vi "Task.vi"() -> ()   [LabVIEW 2015]
uses:
  TASK ERL/List of robots.ctl
  TASK ERL/Status task.ctl
  Zmienne/common msg from UAV-1.vi
  Zmienne/common msg.vi
  Zmienne/Lokalizacja GPS/longitude Quadron.vi
  Zmienne/Lokalizacja GPS/latitude Quadron.vi
  Zmienne/Lokalizacja GPS/latitude.vi
  Zmienne/Lokalizacja GPS/longitude.vi
  Zmienne/Lokalizacja GPS/Longitude Sparus.vi
  Zmienne/Lokalizacja GPS/Latitude Sparus.vi
  Zmienne/Lokalizacja GPS/Latitude dron 1.vi
  Zmienne/Lokalizacja GPS/Longitude dron 1.vi
  Zmienne/Lokalizacja GPS/Longitude dron 2.vi
  Zmienne/Lokalizacja GPS/Latitude dron 2.vi
  TASK ERL/task erl.lvlib
  Zmienne/Lokalizacja GPS/Lokalizacja GPS.lvlib
  <vilib>/Intelligent Energy/WebSockets API/WebSockets/WebSockets.lvlib
  KML/KML.lvlib
  <vilib>/Utility/miscctls.llb/LVStringsAndValuesArrayTypeDef_U16.ctl
  Zmienne/Zmienne.lvlib
panel:
  out "nowa wiadomość":bool
  in  "Tab Control":enum32{"Drone 1", "Sparus"}(tab)
  out "error out 5":errorcluster
  out "sent messages  2":T1
  in  "ROSB WRITE 2":bool
  in  "advertise msg 3":string="{\"op\":\"advertise\", \"topic\":\"common\",\"type\":\"common_msgs/Common\"}"
  in  "rosbridge port 3":u16=9090
  in  "rosbridge server IP 3":string="192.168.1.106"
  out "raw frame 5":string="{\"op\":\"\",\"topic\":\"\",\"Msg\":{\"Sender_name\":\"Raptor\",\"Receiver_name\":\"UGV1-Raptor\",\"Latitude\":0,\"Longitude\":0,\"Value_number\":1,\"status\":\"UGV1-Raptor\"}}"
  in  "STOP ROS WRITE 2":bool
  out "raw frame 4":string="{\"op\":\"\",\"topic\":\"\",\"Msg\":{\"Sender_name\":\"Raptor\",\"Receiver_name\":\"UGV1-Raptor\",\"Latitude\":0,\"Longitude\":0,\"Value_number\":1,\"status\":\"UGV1-Raptor\"}}"
  in  "STOP ROS WRITE":bool
  in  "rosbridge server IP 2":string="192.168.1.68"
  in  "rosbridge port 2":u16=9090
  in  "advertise msg 2":string="{\"op\":\"advertise\", \"topic\":\"common\",\"type\":\"common_msgs/Common\"}"
  in  "ROSB WRITE":bool
  out "error out 4":errorcluster
  out "sent messages":T1
  out "read messages from UAV-1":T1
  in  "Mode 3":bool
  in  "String":string
  in  "Pipe":i32
  out "read messages from AUV sparus":T1
  in  "receiver robot":T2="sparus"
  in  "sender robot":T2="UGV1-Raptor"
  in  "Mode 2":bool
  in  "Additional found item":string="s"
  in  "Status sent between robots":path=path "C:/Users/User/Desktop/ERL 2017/TBM1/Surowe dane/comunnication/Common messages.txt"
  in  "Object recognition":path=path "C:/Users/User/Desktop/ERL 2017/TBM1/Surowe dane/Object recognition/object recognition.txt"
  in  "target ID":string="s"
  in  "... .jpg":string="s"
  in  "found":bool=TRUE
  in  "OPI to find":u16(ring)=3 items=["Underwater - 1 plume (made of 5 orange buoys)"=1, "Underwater - 1 pipe leaks"=2, "Underwater - debris (4 objects)"=3, "Underwater - 1 gate (made of 2 orange buoys)"=4, "Outdoor - 1 Pipe leak on land"=5, "Outdor - second damages on the building wall"=6, "Outdoor - third damages on the building wall"=7, "Indoor - 1 machine room entrance"=8, "Indoor - 1 correct valve (of four valves)"=9]
  out "OPI found":string[][](table)=[["2017-09-19T00:43:17Z", "s", "0,000000", "0,000000", "s", "UGV1-Raptor"], ["2017-09-19T00:43:22Z", "s", "0,000000", "0,000000", "s", "UGV1-Raptor"]]
  in  "Status":T2="Attached"
  in  "Additional status":string="Underwater - debris (4 objects)"
  in  "List of robots":T2="UAV-1"
  in  "Delete":bool
  in  "Number registered subtask":u16(ring)=11 items=["1"=1, "3"=2, "3"=3, "4"=4]
  out "Subtask to do":string[][](table)=[["1", "A1: Outdoors", "", "From the starting point of the building, a ground robot reaches WP5 L within a precision of 3m\navoiding obstacles along the route.", " "], ["2", "A1: Outdoors", "", "A ground robot reaches WP6 L within a precision of 3m with autonomous navigation, avoiding\nobstacles along the route. ", ""], ["3", "A1: Outdoors", "", "The robots recognise the damages outside the building (1 achievement for damage – each damage\ncan only be scored once).", ""], ["4", "A1: Outdoors", "", "The ground robot(s) build(s) an outdoor map of the land pipes area.", ""], ["5", "A1: Outdoors", "", "A ground robot detects the leak marker on the pipe.", ""], ["6", "A1: Outdoors", "", "A ground robot reports which pipe is leaking on land.", ""], ["7", "A1: Outdoors", "", "A ground robot recognises the number on the leaking pipe on land. ", ""], ["8", "A1: Outdoors", "", "Robots localise the unobstructed entrance in real-time in automatic way.", ""], ["9", "A2: Indoors", "", "A ground robot enters inside the building through the unblocked entrance.", ""], ["10", "A2: Indoors", "", "A ground robot finds a safe and unobstructed path to the machine room. (The safe path - collision\nfree from obstacles and structures - from the building entrance to the machine room must be\nshowed on the map).", ""], ["11", "A2: Indoors", "", "The ground robot(s) build a geometric indoor map of the building (Area1). ", ""], ["12", "A2: Indoors", "", "The ground robot(s) build a geometric indoor map of the building (Area2). ", ""], ["13", "A2: Indoors", "", "A ground robot recognises the machine room sign in real-time in automatic way.", ""], ["14", "A2: Indoors", "", "A ground robot enters the machine room", ""], ["15", "A2: Indoors", "", "The ground robot recognises the ID of the correct set of valves in the machine room", ""], ["16", "A2: Indoors", "", "The ground robot closes the correct valve. The robot must close one valve of the set\nautonomously and the other one manually. The process must be recorded by the on board camera\nof the robot.", ""], ["17", "A3: Underwater", "", "The underwater robot provides acoustic and optical images of the gate.", ""], ["18", "A3: Underwater", "", "The underwater robot passes through the gate without touching it. ", ""], ["19", "A3: Underwater", "", "The underwater robot passes through the gate within the first 30 minutes from the start of the run. ", ""], ["20", "A3: Underwater", "", "The underwater robot detects the five plume buoys in real time. Images are needed. ", ""], ["21", "A3: Underwater", "", "The underwater robot recognises the number on the five plume buoys. ", ""], ["22", "A3: Underwater", "", "The underwater robot produces a geometric map of the plume (Area: B1+B2). Father area from\nthe piping assembly", ""], ["23", "A3: Underwater", "", "The underwater robot produces a geometric map of the plume (Area: B3+B4+B5). Closer area to\nthe pipping assembly", ""], ["24", "A3: Underwater", "", "The underwater robot inspects the 4 pipes underwater. ", ""], ["25", "A3: Underwater", "", "The underwater robot detects the leak marker on the pipe in real time. ", ""], ["26", "A3: Underwater", "", "The underwater robot reports which is the number of the leaking pipe by its geometric position. ", ""], ["27", "A3: Underwater", "", "The underwater robot recognises and provides images of the black number stamped on the leaking\npipe", ""], ["28", "A3: Underwater", "", "Following the leaking pipe up to the assembly structure, the underwater robot provides an image\nmosaic of the first half of the leaking pipe. ", ""], ["29", "A3: Underwater", "", "Following the leaking pipe up to the assembly structure, the underwater robot provides an image\nmosaic of the second half of the leaking pipe. ", ""], ["30", "A3: Underwater", "", "The underwater robot provides a 3D reconstruction of the manipulation console where the correct\nunderwater valve is. ", ""], ["31", "A3: Underwater", "", "The underwater robot closes the correct valve with a rotation of the first 45 degrees. The process\nmust be recorded by the on board camera of the robot. ", ""], ["32", "A3: Underwater", "", "The underwater robot closes the correct valve with a rotation of the last 45 degrees (the process\nmust be recorded by the on board camera of the robot).", ""], ["33", "A4: Cooperation", "", "The underwater robot communicates through a surface robot or directly to the ground robot the\nfound leaking pipe.", ""], ["34", "A4: Cooperation", "", "The ground robot receives and decodes the message with the correct leaking pipe sent by directly\nby the underwater or through the surface robot. ", ""], ["35", "A4: Cooperation", "", "The ground robot communicates the correct land leaking pipe to the underwater robot (directly or\nthrough the surface robot). ", ""], ["36", "A4: Cooperation", "", "The underwater robot receives and decodes the message with the correct land leaking pipe sent by\nthe ground robot or the surface robot", ""], ["37", "A4: Cooperation", "", "The ground robot and the underwater robot close the correct valves in a synchronised process.", ""]]
  in  "Add leaking pipe":bool
  out "Status sent between robots and control station":string[][](table)
  in  "Cancel":bool
  in  "Setup":bool=TRUE
  in  "Done":bool=TRUE
  in  "Start":bool=TRUE
  in  "Ready":bool
  in  "stop":bool=TRUE
  out "Subtask registered event":string[][](table)
  in  "Subtask":u16(ring)=2
  out "All Subtask Status":string[][](table)=[["1", "A1: Outdoors", "", "From the starting point of the building, a ground robot reaches WP5 L within a precision of 3m\navoiding obstacles along the route.", " "], ["2", "A1: Outdoors", "", "A ground robot reaches WP6 L within a precision of 3m with autonomous navigation, avoiding\nobstacles along the route. ", ""], ["3", "A1: Outdoors", "", "The robots recognise the damages outside the building (1 achievement for damage – each damage\ncan only be scored once).", ""], ["4", "A1: Outdoors", "", "The ground robot(s) build(s) an outdoor map of the land pipes area.", ""], ["5", "A1: Outdoors", "", "A ground robot detects the leak marker on the pipe.", ""], ["6", "A1: Outdoors", "", "A ground robot reports which pipe is leaking on land.", ""], ["7", "A1: Outdoors", "", "A ground robot recognises the number on the leaking pipe on land. ", ""], ["8", "A1: Outdoors", "", "Robots localise the unobstructed entrance in real-time in automatic way.", ""], ["9", "A2: Indoors", "", "A ground robot enters inside the building through the unblocked entrance.", ""], ["10", "A2: Indoors", "", "A ground robot finds a safe and unobstructed path to the machine room. (The safe path - collision\nfree from obstacles and structures - from the building entrance to the machine room must be\nshowed on the map).", ""], ["11", "A2: Indoors", "", "The ground robot(s) build a geometric indoor map of the building (Area1). ", ""], ["12", "A2: Indoors", "", "The ground robot(s) build a geometric indoor map of the building (Area2). ", ""], ["13", "A2: Indoors", "", "A ground robot recognises the machine room sign in real-time in automatic way.", ""], ["14", "A2: Indoors", "", "A ground robot enters the machine room", ""], ["15", "A2: Indoors", "", "The ground robot recognises the ID of the correct set of valves in the machine room", ""], ["16", "A2: Indoors", "", "The ground robot closes the correct valve. The robot must close one valve of the set\nautonomously and the other one manually. The process must be recorded by the on board camera\nof the robot.", ""], ["17", "A3: Underwater", "", "The underwater robot provides acoustic and optical images of the gate.", ""], ["18", "A3: Underwater", "", "The underwater robot passes through the gate without touching it. ", ""], ["19", "A3: Underwater", "", "The underwater robot passes through the gate within the first 30 minutes from the start of the run. ", ""], ["20", "A3: Underwater", "", "The underwater robot detects the five plume buoys in real time. Images are needed. ", ""], ["21", "A3: Underwater", "", "The underwater robot recognises the number on the five plume buoys. ", ""], ["22", "A3: Underwater", "", "The underwater robot produces a geometric map of the plume (Area: B1+B2). Father area from\nthe piping assembly", ""], ["23", "A3: Underwater", "", "The underwater robot produces a geometric map of the plume (Area: B3+B4+B5). Closer area to\nthe pipping assembly", ""], ["24", "A3: Underwater", "", "The underwater robot inspects the 4 pipes underwater. ", ""], ["25", "A3: Underwater", "", "The underwater robot detects the leak marker on the pipe in real time. ", ""], ["26", "A3: Underwater", "", "The underwater robot reports which is the number of the leaking pipe by its geometric position. ", ""], ["27", "A3: Underwater", "", "The underwater robot recognises and provides images of the black number stamped on the leaking\npipe", ""], ["28", "A3: Underwater", "", "Following the leaking pipe up to the assembly structure, the underwater robot provides an image\nmosaic of the first half of the leaking pipe. ", ""], ["29", "A3: Underwater", "", "Following the leaking pipe up to the assembly structure, the underwater robot provides an image\nmosaic of the second half of the leaking pipe. ", ""], ["30", "A3: Underwater", "", "The underwater robot provides a 3D reconstruction of the manipulation console where the correct\nunderwater valve is. ", ""], ["31", "A3: Underwater", "", "The underwater robot closes the correct valve with a rotation of the first 45 degrees. The process\nmust be recorded by the on board camera of the robot. ", ""], ["32", "A3: Underwater", "", "The underwater robot closes the correct valve with a rotation of the last 45 degrees (the process\nmust be recorded by the on board camera of the robot).", ""], ["33", "A4: Cooperation", "", "The underwater robot communicates through a surface robot or directly to the ground robot the\nfound leaking pipe.", ""], ["34", "A4: Cooperation", "", "The ground robot receives and decodes the message with the correct leaking pipe sent by directly\nby the underwater or through the surface robot. ", ""], ["35", "A4: Cooperation", "", "The ground robot communicates the correct land leaking pipe to the underwater robot (directly or\nthrough the surface robot). ", ""], ["36", "A4: Cooperation", "", "The underwater robot receives and decodes the message with the correct land leaking pipe sent by\nthe ground robot or the surface robot", ""], ["37", "A4: Cooperation", "", "The ground robot and the underwater robot close the correct valves in a synchronised process.", ""]]
  in  "Subtask registered eveny":path=path "C:/Users/User/Desktop/ERL 2017/TBM1/Surowe dane/Subtask registered event.txt"
  in  "Mode":bool
  # "Manual"
  # "Autonomous"
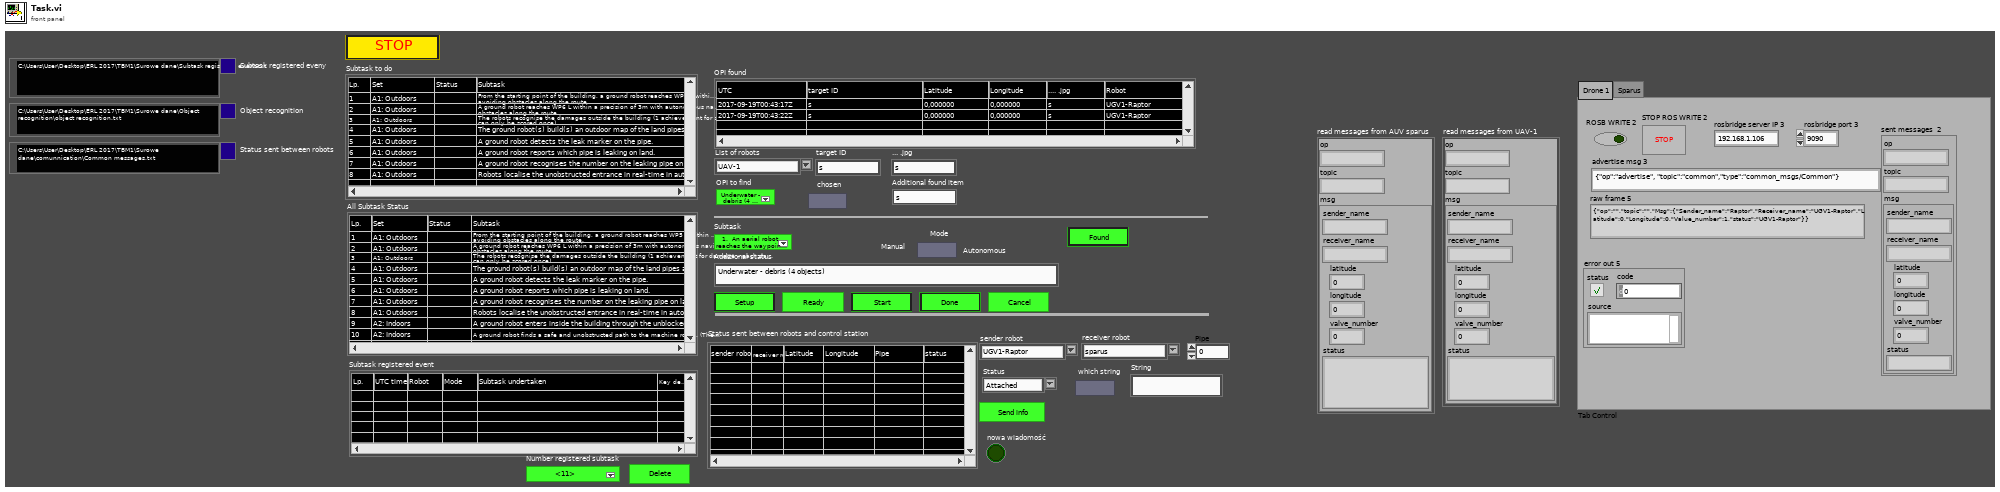
[diagram p1: front panel]
types:
  T1 = cluster{"op":string, "topic":string, "msg":cluster{"sender_name":string, "receiver_name":string, "latitude":dbl, "longitude":dbl, "valve_number":i32, "status":string}}
  T2 = typedef "Biblioteka moduł map v3.lvlib/task erl.lvlib/List of robots.ctl" = string
  T3 = cluster{"AUV-Sparus":cluster{"Navigation data":string[][], "Data sampling frequency":string}, "UAV-1":cluster{"Navigation data":string[][], "Data sampling frequency":string}, "UAV-2":cluster{"Navigation data":string[][], "Data sampling frequency":string}, "UGV1-Raptor":cluster{"Navigation data":string[][], "Data sampling frequency":string}, "UGV2-Quadron":cluster{"Navigation data":string[][], "Data sampling frequency":string}}
  T4 = typedef "LVStringsAndValuesArrayTypeDef_U16.ctl" = cluster{"String":string, "Value":u16}[]
  T5 = typedef "Biblioteka moduł map v3.lvlib/task erl.lvlib/Status task.ctl" = string
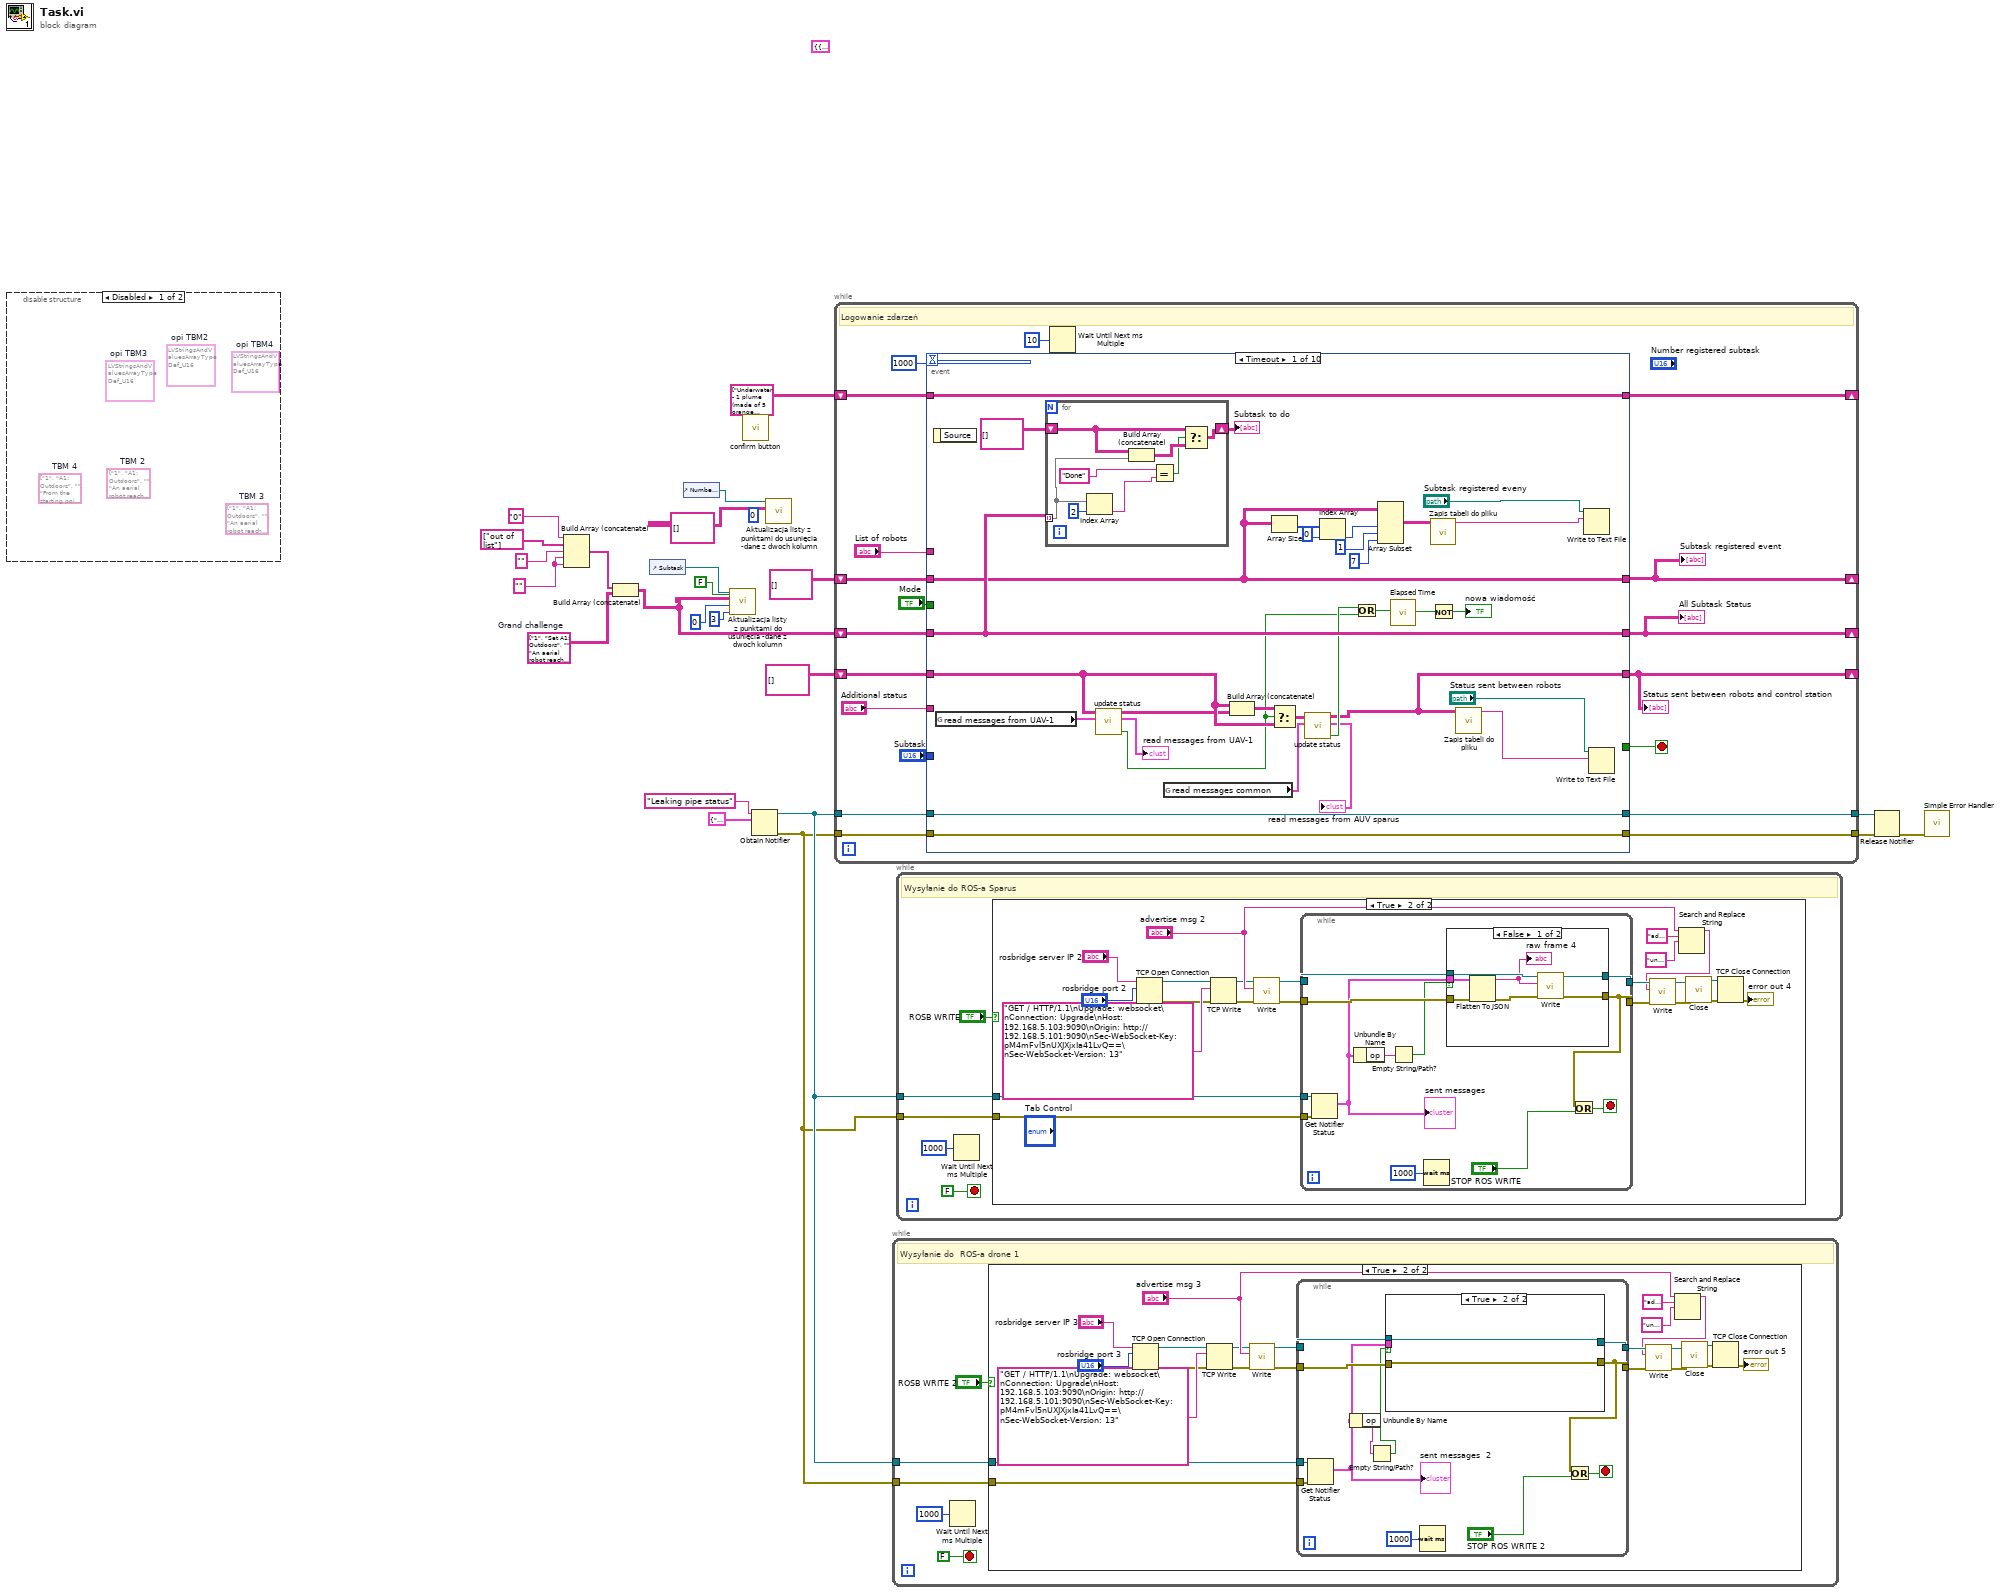
[diagram p0: block diagram]
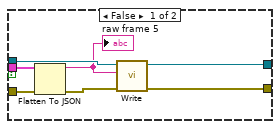
[diagram p3: hidden frame]
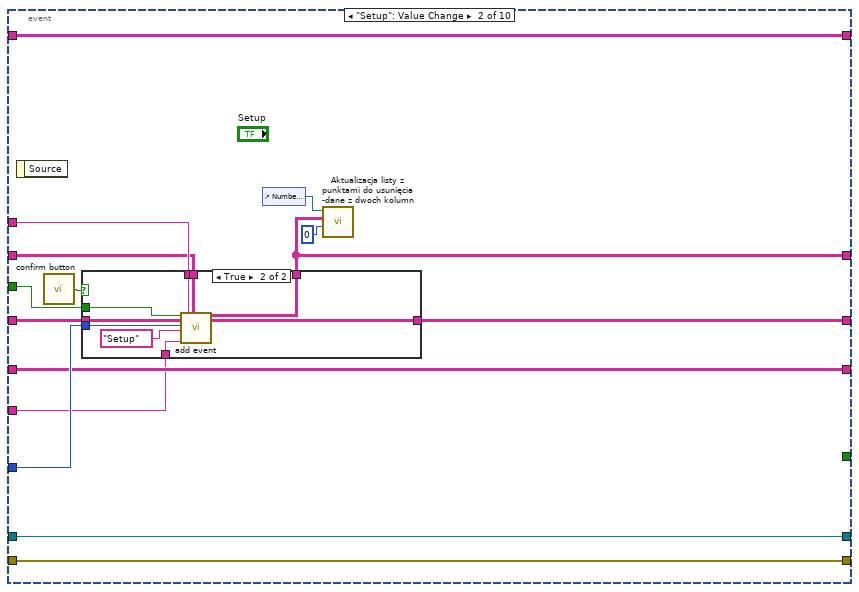
[diagram p7: hidden frame]
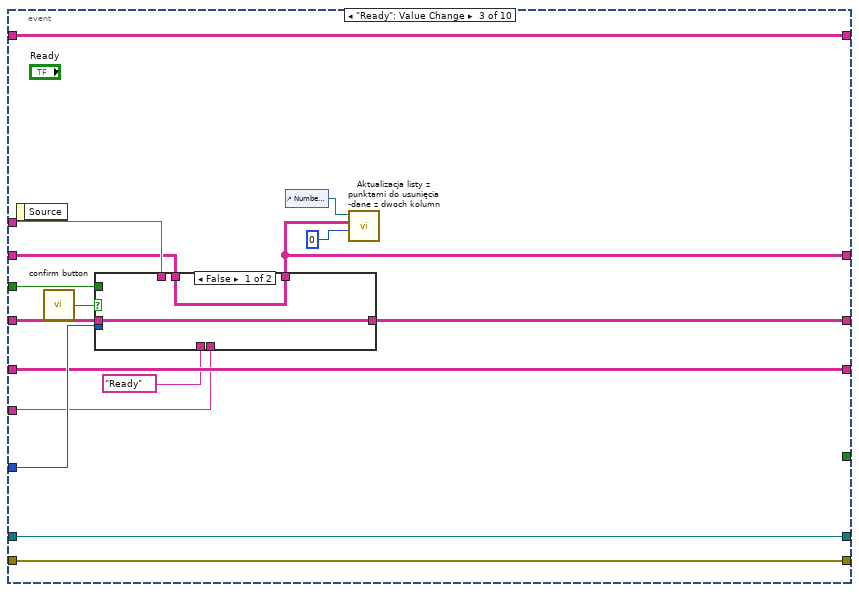
[diagram p9: hidden frame]
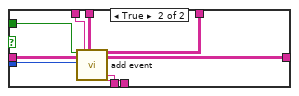
[diagram p10: hidden frame]
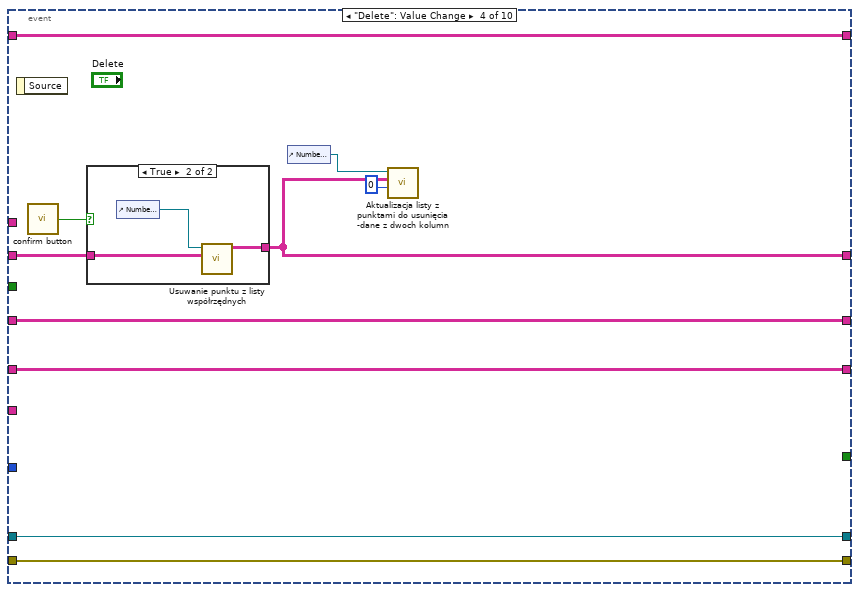
[diagram p11: hidden frame]
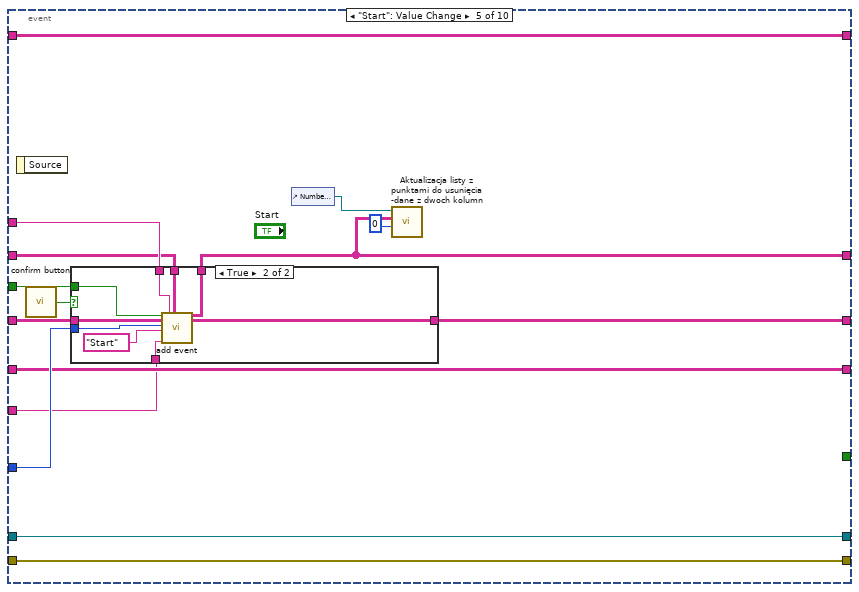
[diagram p13: hidden frame]
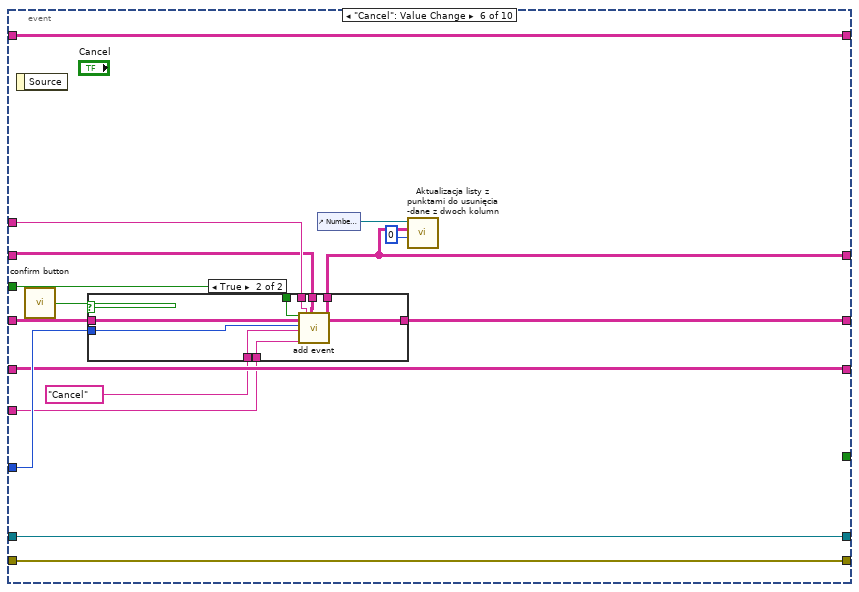
[diagram p15: hidden frame]
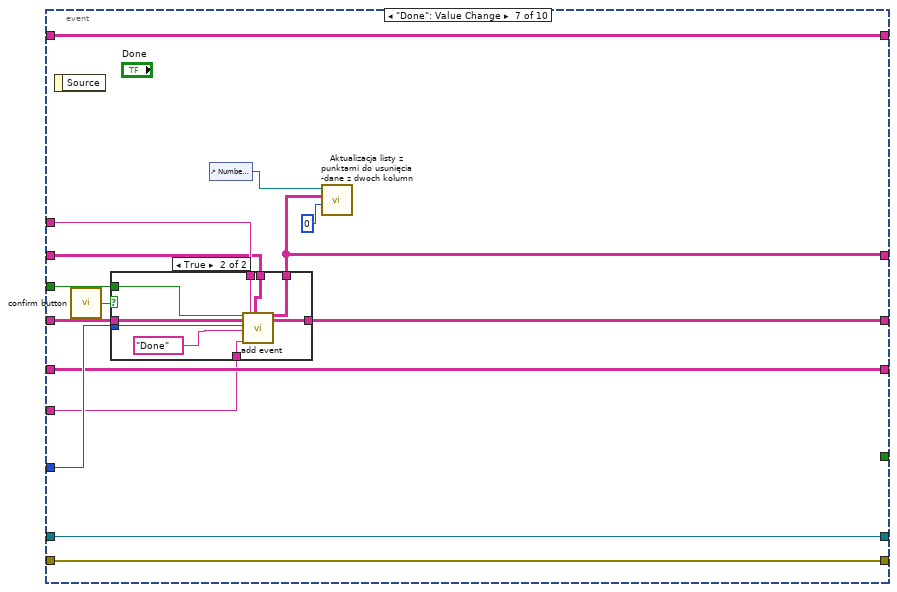
[diagram p17: hidden frame]
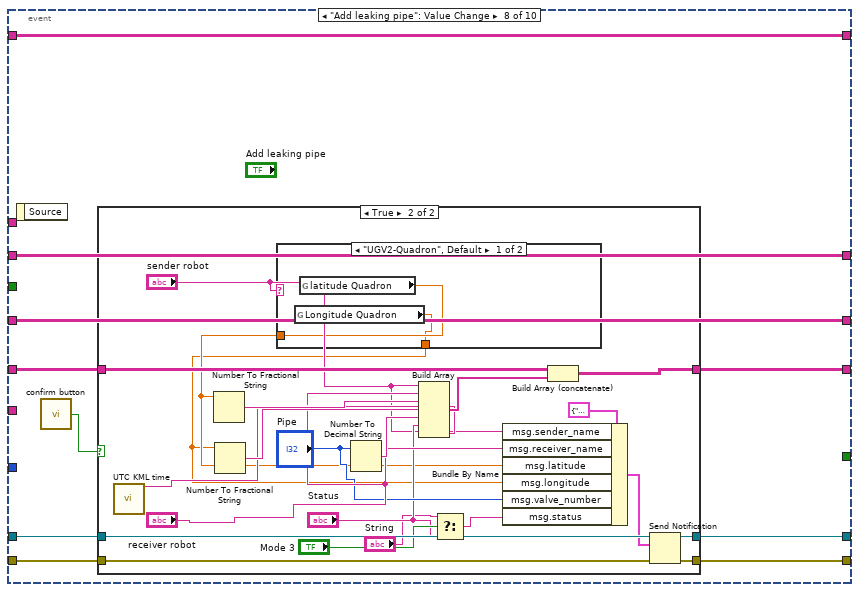
[diagram p19: hidden frame]
diagram:
  w3 = string[][] [["1", "Set A1: Outdoors", "", "An aerial robot reaches the waypoints WP1 A within a radius of 5 m in autonomous navigation."], ["2", "Set A1: Outdoors", "", "An aerial robot reaches the waypoints WP2 A within a radius of 5 m in autonomous navigation."], ["3", "Set A1: Outdoors", "", "An aerial robot reaches the waypoints WP3 A within a radius of 5 m in autonomous navigation."], ["4", "Set A1: Outdoors", "", "A ground robot reaches the waypoints WP1 L within a precision of 3m."], ["5", "Set A1: Outdoors", "", "A ground robot reaches the waypoints WP2 L within a precision of 3m."], ["6", "Set A1: Outdoors", "", "A ground robot reaches the waypoints WP5 L within a precision of 3m."], ["7", "Set A1: Outdoors", "", "A ground robot reaches the WP3 L within a precision of 3 m in autonomous navigation."], ["8", "Set A1: Outdoors", "", "A ground robot reaches the WP4 L within a precision of 3 m in autonomous navigation."], ["9", "Set A1: Outdoors", "", "A ground robot reaches the WP6 L within a precision of 3 m in autonomous navigation."], ["10", "Set A1: Outdoors", "", "Within 30 minutes of start of the run, a robot reports the correct location (within radius 5 m) of the missing worker outside the building. "], ["11", "Set A1: Outdoors", "", "An aerial robot deploys the first-aid kit (within radius 2 m) from the worker outside the building"], ["12", "Set A1: Outdoors", "", "The aerial robot transfers the first-aid kit to the land robot outside the building. (It must be directly deployed on the platform or within a radius of 1 m from it) "], ["13", "Set A1: Outdoors", "", "Robots reports the damages on the land pipes. D1"], ["14", "Set A1: Outdoors", "", "Robots reports the damages on the land pipes. D2"], ["15", "Set A1: Outdoors", "", "Robots reports the damages on the land pipes. D3"], ["16", "Set A1: Outdoors", "", "A robot detects the leak marker on the pipe."], ["17", "Set A1: Outdoors", "", "A robot reports the pipe that is leaking on land. "], ["18", "Set A1: Outdoors", "", "A robot recognises the number on the leaking pipe on land. "], ["19", "Set A1: Outdoors", "", "The robots recognise the damages on the wall of the building.  D1"], ["20", "Set A1: Outdoors", "", "The robots recognise the damages on the wall of the building.  D2"], ["21", "Set A1: Outdoors", "", "The robots recognise the damages on the wall of the building.  D3"], ["22", "Set A1: Outdoors", "", "A robot localises the unobstructed entrance in real-time in automatic way."], ["23", "Set A1: Outdoors", "", "Robots localise the obstructed entrances. E1"], ["24", "Set A1: Outdoors", "", "Robots localise the obstructed entrances. E2"], ["25", "Set A1: Outdoors", "", "Robots find a safe and unobstructed path to the unblocked entry of the building for a ground robot. (The path is shown on the map). "], ["26", "Set A1: Outdoors", "", "From the starting point, a ground robot follows a safe path (collision free from obstacles and structures) to the unobstructed building entrance."], ["27", "Set A1: Outdoors", "", "The aerial robot builds a 2D or 3D map of the designated vertical wall "], ["28", "Set A1: Outdoors", "", "The aerial robot builds the map on board during the flight. The map must be shown to the referees just after the flight finishes. "], ["29", "Set A1: Outdoors", "", "Robots build an outdoor map of the land pipes area with OPIs (North-West side)."], ["30", "Set A1: Outdoors", "", "Robots build an outdoor map of the land pipes area with OPIs (North-East side)."], ["31", "Set A1: Outdoors", "", "Robots build an outdoor map of the land pipes area with OPIs (South-West side)."], ["32", "Set A1: Outdoors", "", "Robots build an outdoor map of the land pipes area with OPIs (South-East side)."], ["33", "Set A2: Indoors", "", "A ground robot enters the building through the unobstructed door"], ["34", "Set A2: Indoors", "", "Within 30 minutes of start of the run, a ground robot reports the correct location of the missing worker inside the building. "], ["35", "Set A2: Indoors", "", "The missing worker is detected in real-time in an automatic way. "], ["36", "Set A2: Indoors", "", "A ground robot deploys the first-aid kit (within radius 1 m) from the worker inside the building. \n"], ["37", "Set A2: Indoors", "", "The ground robot(s) recognise the damages on the wall of the building.  D1"], ["38", "Set A2: Indoors", "", "The ground robot(s) recognise the damages on the wall of the building.  D2"], ["39", "Set A2: Indoors", "", "From the building entrance, a ground robot follows a safe path (collision free from obstacles and structures) to the machine room. "], ["40", "Set A2: Indoors", "", "A ground robot recognises the machine room sign in real-time and in automatic way."], ["41", "Set A2: Indoors", "", "A ground robot enters the machine room. "], ["42", "Set A2: Indoors", "", "The ground robot(s) builds a geometric indoor map of the building.  Area 1"], ["43", "Set A2: Indoors", "", "The ground robot(s) builds a geometric indoor map of the building.  Area 2"], ["44", "Set A2: Indoors", "", "A ground robot recognises the ID of the correct set of valves in the machine room."], ["45", "Set A2: Indoors", "", "A ground robot closes the correct valve manual."], ["46", "Set A2: Indoors", "", "A ground robot closes the correct valve autonomous."], ["47", "Set A3: Underwater", "", "The underwater robot provides images of the gate. Acoustic buoy-1"], ["48", "Set A3: Underwater", "", "The underwater robot provides images of the gate. Acoustic buoy-2 "], ["49", "Set A3: Underwater", "", "The underwater robot provides images of the gate. Optical buoy-1"], ["50", "Set A3: Underwater", "", "The underwater robot provides images of the gate. Optical buoy-2"], ["51", "Set A3: Underwater", "", "The underwater robot detects the plume buoys in real time. Images are needed.  B1"], ["52", "Set A3: Underwater", "", "The underwater robot detects the plume buoys in real time. Images are needed.  B2"], ["53", "Set A3: Underwater", "", "The underwater robot detects the plume buoys in real time. Images are needed.  B3"], ["54", "Set A3: Underwater", "", "The underwater robot detects the plume buoys in real time. Images are needed.  B4"], ["55", "Set A3: Underwater", "", "The underwater robot detects the plume buoys in real time. Images are needed.  B5"], ["56", "Set A3: Underwater", "", "The underwater robot recognises the number on the plume buoys B1"], ["57", "Set A3: Underwater", "", "The underwater robot recognises the number on the plume buoys B2"], ["58", "Set A3: Underwater", "", "The underwater robot recognises the number on the plume buoys B3"], ["59", "Set A3: Underwater", "", "The underwater robot recognises the number on the plume buoys B4"], ["60", "Set A3: Underwater", "", "The underwater robot recognises the number on the plume buoys B5"], ["61", "Set A3: Underwater", "", "The underwater robot produces a geometric map of the plume (Area: B1+B2)."], ["62", "Set A3: Underwater", "", "The underwater robot produces a geometric map of the plume (Area: B3+B4+B5)."], ["63", "Set A3: Underwater", "", "The underwater robot detects the leak marker on the pipe in real time. "], ["64", "Set A3: Underwater", "", "The underwater robot recognises and provides images of the black number stamped on the leaking pipe."], ["65", "Set A3: Underwater", "", "The underwater robot reports which is the number of the leaking pipe by its geometric position. "], ["66", "Set A3: Underwater", "", "The underwater robot inspects the four pipes underwater. Provide images.1"], ["67", "Set A3: Underwater", "", "The underwater robot inspects the four pipes underwater. Provide images.2"], ["68", "Set A3: Underwater", "", "The underwater robot inspects the four pipes underwater. Provide images.3"], ["69", "Set A3: Underwater", "", "The underwater robot inspects the four pipes underwater. Provide images.4"], ["70", "Set A3: Underwater", "", "Following the leaking pipe up to the assembly structure, the underwater robot provides an image mosaic of the first half of the leaking pipe."], ["71", "Set A3: Underwater", "", "Following the leaking pipe up to the assembly structure, the underwater robot provides an image mosaic of the second half of the leaking pipe. "], ["72", "Set A3: Underwater", "", "The underwater robot provides images of the structure sides.  North"], ["73", "Set A3: Underwater", "", "The underwater robot provides images of the structure sides.  South"], ["74", "Set A3: Underwater", "", "The underwater robot provides images of the structure sides.  East"], ["75", "Set A3: Underwater", "", "The underwater robot provides images of the structure sides.  West"], ["76", "Set A3: Underwater", "", "The underwater robot provides a 3D reconstruction of the structure. "], ["77", "Set A3: Underwater", "", "The underwater robot localises the missing worker underwater within a radius of 5 meters."], ["78", "Set A3: Underwater", "", "The underwater robot gives the dimensions and geometrical shape of the closest object to the worker"], ["79", "Set A3: Underwater", "", "The underwater robot provides 3D reconstruction of the worker."], ["80", "Set A3: Underwater", "", "The underwater robot provides a 2D acoustic or optical map of the debris.  Area 1"], ["81", "Set A3: Underwater", "", "The underwater robot provides a 2D acoustic or optical map of the debris.  Area 2"], ["82", "Set A3: Underwater", "", "The underwater robot provides a 3D reconstruction of the manipulation console where the correct underwater valve is. "], ["83", "Set A3: Underwater", "", "The underwater robot closes the correct valve with a rotation of the first 45 degrees. The process must be recorded by the on board camera of the robot"], ["84", "Set A3: Underwater", "", "The underwater robot closes the correct valve with a rotation of the last 45 degrees.  The process must be recorded by the on board camera of the robot."], ["85", "Set A4: Cooperation", "", "The underwater robot communicates the correct underwater leaking pipe to the aerial or ground robot. Directly or through the surface robot."], ["86", "Set A4: Cooperation", "", "The aerial or ground robot receives and decodes the message with the correct leaking pipe sent by directly by the underwater or through the surface robot."], ["87", "Set A4: Cooperation", "", "The aerial or ground robot communicates the correct land leaking pipe to the underwater robot (directly or through the surface robot)."], ["88", "Set A4: Cooperation", "", "The underwater robot receives and decodes the message with the correct land leaking pipe sent by the aerial or ground robot (directly or through the surface robot)."], ["89", "Set A4: Cooperation", "", "The ground robot and the underwater robot close the correct valves in a synchronised process. "], ["90", "Set A4: Cooperation", "", "The aerial robot communicates to the ground robot the safe path to the building"], ["91", "Set A5: General", "", "The ground robots return to the landing area once all the tasks have been done"], ["92", "Set A5: General", "", "The underwater robot surfaces in a controlled way once all the tasks have been done."], ["93", "Set A5: General", "", "The aerial robots return to the landing area once all the tasks have been done. "], ["94", "Set A5: General", "", "The ground robot(s) transmits live position and images/video to the control station during the run. "], ["95", "Set A5: General", "", "The aerial robot(s) transmits live position and images/video to the control station during the run. "], ["96", "Set A5: General", "", "The marine robot(s) transmits live position and images/video to the control station during the run or the manipulation task."]]  # Grand challenge
  w10 = ""
  (unwired) T3 {"AUV-Sparus"={"Navigation data"=[], "Data sampling frequency"=""}, "UAV-1"={"Navigation data"=[], "Data sampling frequency"=""}, "UAV-2"={"Navigation data"=[], "Data sampling frequency"=""}, "UGV1-Raptor"={"Navigation data"=[], "Data sampling frequency"=""}, "UGV2-Quadron"={"Navigation data"=[], "Data sampling frequency"=""}} ("Vehicle navigation data")
  (unwired) 0 ("text add 1")
  n1 = disable-structure shown="Disabled" {
    frame Disabled {
      (unwired) string[][] [["1", "A1: Outdoors", "", "An aerial robot reaches WP1A, WP2A, WP3A, within a radius of 5 meters with autonomous\nnavigation. Waypoints can be reached in no specific order and the team can suggest additional\nwaypoints to their flight plan.", " "], ["2", "A1: Outdoors", "", "Within first 30 minutes of the start of the run, an aerial robot reports correct location (within\nradius of 5 m) of the missing worker on land.", ""], ["3", "A1: Outdoors", "", "An aerial robot deploys the first-aid kit within a radius of 2 m from the worker found on land", ""], ["4", "A1: Outdoors", "", "An aerial robot reports which pipe(s) are damaged on land (one achievement per damage).", ""], ["5", "A1: Outdoors", "", "An aerial robot detects the leak marker on the pipe.", ""], ["6", "A1: Outdoors", "", "An aerial robot reports which pipe is leaking on land", ""], ["7", "A1: Outdoors", "", "The aerial robot builds an outdoor map of the land pipes area with OPIs (North-West side). Use\nthe information from each robot to provide only one map.", ""], ["8", "A1: Outdoors", "", "The aerial robot builds an outdoor map of the land pipes area with OPIs (North-East side). Use\nthe information from each robot to provide only one map.", ""], ["9", "A1: Outdoors", "", "The aerial robot builds an outdoor map of the land pipes area with OPIs (South-West side). Use\nthe information from each robot to provide only one map.", ""], ["10", "A1: Outdoors", "", "The aerial robot builds an outdoor map of the land pipes area with OPIs (South-East side). Use\nthe information from each robot to provide only one map.", ""], ["11", "A1: Outdoors", "", "The aerial robot builds the maps on board during the flight. The maps must be shown to the\nreferees just after the flight finishes. ", ""], ["12", "Set A2: Underwater", "", "The underwater robot provides acoustic and optical images of the gate.", ""], ["13", "Set A2: Underwater", "", "The underwater robot passes through the gate without touching it. ", ""], ["14", "Set A2: Underwater", "", "The underwater robot passes through the gate within the first 30 minutes from the start of the run. ", ""], ["15", "Set A2: Underwater", "", "The underwater robot detects the five plume buoys in real time. Images are needed. ", ""], ["16", "Set A2: Underwater", "", "The underwater robot recognises the number on the five plume buoys. ", ""], ["17", "Set A2: Underwater", "", "The underwater robot produces a geometric map of the plume (Area: B1+B2). Father area from\nthe piping assembly.", ""], ["18", "Set A2: Underwater", "", "The underwater robot produces a geometric map of the plume (Area: B3+B4+B5). Closer area to\nthe pipping assembly", ""], ["19", "Set A2: Underwater", "", "The underwater robot detects the leak marker on the pipe in real time. ", ""], ["20", "Set A2: Underwater", "", "The underwater robot recognises and provides images of the black number stamped on the leaking\npipe.", ""], ["21", "Set A2: Underwater", "", "The underwater robot reports which is the number of the leaking pipe by its geometric position. ", ""], ["22", "Set A2: Underwater", "", "Following the leaking pipe up to the assembly structure, the underwater robot provides an image\nmosaic of the first half of the leaking pipe. ", ""], ["23", "Set A2: Underwater", "", "Following the leaking pipe up to the assembly structure, the underwater robot provides an image\nmosaic of the second half of the leaking pipe. ", ""], ["24", "Set A2: Underwater", "", "The underwater robot provides images of the structure sides (North, South, East and West).", ""], ["25", "Set A2: Underwater", "", "The underwater robot provides a 3D reconstruction of the structure (front and rear).", ""], ["26", "Set A2: Underwater", "", "The underwater robot provides a 2D acoustic or optical map of the debris (Area 1 and Area 2", ""], ["27", "Set A2: Underwater", "", "The underwater robot localises the missing worker underwater within a radius of 5 meters.\nProvide images and latitude/longitude.", ""], ["28", "Set A2: Underwater", "", "The underwater robot gives the dimensions and geometrical shape of the closest object to the\nworker", ""], ["29", "Set A2: Underwater", "", "The underwater robot provides 3D reconstruction of the worker.", ""], ["30", "Set A2: Underwater", "", "The underwater robot surfaces within a radius of 2 meters from the worker position.", ""], ["31", "Set A3: Cooperation", "", "The underwater robot communicates directly or through a surface robot to the aerial robot the\nposition of the underwater worker (within a radius of 5 meters).", ""], ["32", "Set A3: Cooperation", "", "The aerial robot receives and decodes the message with the position of the worker sent by the\nunderwater/surface robot.", ""], ["33", "Set A3: Cooperation", "", "The aerial robot, upon receiving the position of the underwater worker, takes a picture (from the\nauthorised aerial volume) of the harbour area showing either the underwater robot or the surface\nrobot on the position that marks where the worker is. (The image includes location).", ""], ["34", "Set A3: Cooperation", "", "The underwater robot communicates the correct underwater leaking pipe to the aerial robot. ", ""], ["35", "Set A3: Cooperation", "", "The aerial robot receives and decodes the message with the correct leaking pipe sent by directly\nby the underwater or through the surface robot. ", ""], ["36", "Set A3: Cooperation", "", "The aerial robot communicates the correct land leaking pipe to the underwater robot (directly or\nthrough the surface robot). ", ""], ["37", "Set A3: Cooperation", "", "The underwater robot receives and decodes the message with the correct land leaking pipe sent by\nthe aerial robot or the surface robot.", ""], ["38", "Set A4: General", "", "The aerial robots return to the landing area once all the tasks have been done. ", ""], ["39", "Set A4: General", "", "The underwater robot surfaces in a controlled way once all the tasks have been done.", ""], ["40", "Set A4: General", "", "Benchmarking data is delivered appropriately (time and format)", ""], ["41", "Set A4: General", "", "The aerial robot(s) transmits live position and images/video to the control station during the run", ""], ["42", "Set A4: General", "", "The marine robot(s) transmits live position and images/video to the control station during the run\nor the manipulation task.", ""]]  # TBM 3
      (unwired) string[][] [["1", "A1: Outdoors", "", "An aerial robot reaches WP1A, WP2A, WP3A, within a radius of 5 meters with autonomous\nnavigation. Waypoints can be reached in no specific order and the team can suggest additional\nwaypoints to their flight plan.", " "], ["2", "A1: Outdoors", "", "A ground robot reaches WP1L with a precision of 3 m.", ""], ["3", "A1: Outdoors", "", "A ground robot reaches WP2 L with a precision of 3 m.", ""], ["4", "A1: Outdoors", "", "A ground robot reaches WP3 L within a precision of 3 m in autonomous navigation.", ""], ["5", "A1: Outdoors", "", "A ground robot reaches land piping area WP4 L within a precision of 3 m in autonomous\nnavigation.", ""], ["6", "A1: Outdoors", "", "Within first 30 minutes of the start of the run, a robot reports correct location (within radius of 5\nm) of the missing worker outside the building.", ""], ["7", "A1: Outdoors", "", "An aerial robot deploys the first-aid kit within a radius of 2 m from the worker found on land\noutside the building.", ""], ["8", "A1: Outdoors", "", "An aerial robot transfers the first-aid kit to the land robot outside the building. (It must be directly\ndeployed on the platform or within a radius of 1 m from it).", ""], ["9", "A1: Outdoors", "", "Robots recognise the damages outside the building (1 achievement for damage – each damage can\nonly be scored once).", ""], ["10", "A1: Outdoors", "", "Robots localise the unobstructed entrance in an automatic way", ""], ["11", "A1: Outdoors", "", "Robots localise the obstructed entrances.", ""], ["12", "A1: Outdoors", "", "Robots find a safe and unobstructed path to the unblocked entry of the building for the ground\nrobot (the safe path - collision free from obstacles and structures - from the starting point to the\nunobstructed building entrance must be showed on the map).", ""], ["13", "A1: Outdoors", "", "Robots build an outdoor map of the land pipes area with OPIs (North-West side). Use the\ninformation from each domain and from each robot to provide only one map.", ""], ["14", "A1: Outdoors", "", "Robots build an outdoor map of the land pipes area with OPIs (North-East side).Use the\ninformation from each domain and from each robot to provide only one map.", ""], ["15", "A1: Outdoors", "", "Robots build an outdoor map of the land pipes area with OPIs (South-West side). Use the\ninformation from each domain and from each robot to provide only one map.", ""], ["16", "A1: Outdoors", "", "Robots build an outdoor map of the land pipes area with OPIs (South-East side).Use the\ninformation from each domain and from each robot to provide only one map.", ""], ["17", "A2: Indoors", "", "A ground robot enters the building", ""], ["18", "A2: Indoors", "", "Within first 30 minutes of the start of the run, a ground robot reports correct location of missing\nworker inside the building.", ""], ["19", "A2: Indoors", "", "The missing worker is detected in real-time in an automatic way.", ""], ["20", "A2: Indoors", "", "A ground robot deploys the first-aid kit within a radius of 1 m from the worker found inside the\nbuilding.", ""], ["21", "A2: Indoors", "", "The ground robot(s) recognise the damages inside the building (1 achievement for damage – each\ndamage can only be scored once).", ""], ["22", "A2: Indoors", "", "A ground robot finds a safe and unobstructed path to the machine room. (The safe path - collision\nfree from obstacles and structures - from the building entrance to the machine room must be\nshowed on the map).", ""], ["23", "A2: Indoors", "", "A ground robot recognizes the machine room sign in real-time and in automatic way.", ""], ["24", "A2: Indoors", "", "A ground robot enters the machine room.", ""], ["25", "A2: Indoors", "", "The ground robot(s) build a geometric indoor map of the building (Area1). (Use the best map or a\ncombination of ground robots maps)", ""], ["26", "A2: Indoors", "", "The ground robot(s) build a geometric indoor map of the building (Area2). (Use the best map or a\ncombination of ground robots maps).", ""], ["27", "A3: Cooperation", "", "The aerial robot communicates to the land robot the safe path to the building.", ""], ["28", "A4: General", "", "The aerial robots return to the landing area once all the tasks have been done. ", ""], ["29", "A4: General", "", "The ground robots return to the landing area all the tasks have been done.", ""], ["30", "A4: General", "", "Benchmarking data is delivered appropriately (time and format)", ""], ["31", "A4: General", "", "The ground robot(s) transmits live position and images/video to the control station during the run.", ""], ["32", "A4: General", "", "The aerial robot(s) transmits live position and images/video to the control station during the run.", ""]]  # TBM 2
      (unwired) string[][] [["1", "A1: Outdoors", "", "From the starting point of the building, a ground robot reaches WP5 L within a precision of 3m\navoiding obstacles along the route.", " "], ["2", "A1: Outdoors", "", "A ground robot reaches WP6 L within a precision of 3m with autonomous navigation, avoiding\nobstacles along the route. ", ""], ["3", "A1: Outdoors", "", "The robots recognise the damages outside the building (1 achievement for damage – each damage\ncan only be scored once).", ""], ["4", "A1: Outdoors", "", "The ground robot(s) build(s) an outdoor map of the land pipes area.", ""], ["5", "A1: Outdoors", "", "A ground robot detects the leak marker on the pipe.", ""], ["6", "A1: Outdoors", "", "A ground robot reports which pipe is leaking on land.", ""], ["7", "A1: Outdoors", "", "A ground robot recognises the number on the leaking pipe on land. ", ""], ["8", "A1: Outdoors", "", "Robots localise the unobstructed entrance in real-time in automatic way.", ""], ["9", "A2: Indoors", "", "A ground robot enters inside the building through the unblocked entrance.", ""], ["10", "A2: Indoors", "", "A ground robot finds a safe and unobstructed path to the machine room. (The safe path - collision\nfree from obstacles and structures - from the building entrance to the machine room must be\nshowed on the map).", ""], ["11", "A2: Indoors", "", "The ground robot(s) build a geometric indoor map of the building (Area1). ", ""], ["12", "A2: Indoors", "", "The ground robot(s) build a geometric indoor map of the building (Area2). ", ""], ["13", "A2: Indoors", "", "A ground robot recognises the machine room sign in real-time in automatic way.", ""], ["14", "A2: Indoors", "", "A ground robot enters the machine room", ""], ["15", "A2: Indoors", "", "The ground robot recognises the ID of the correct set of valves in the machine room", ""], ["16", "A2: Indoors", "", "The ground robot closes the correct valve. The robot must close one valve of the set\nautonomously and the other one manually. The process must be recorded by the on board camera\nof the robot.", ""], ["17", "A3: Underwater", "", "The underwater robot provides acoustic and optical images of the gate.", ""], ["18", "A3: Underwater", "", "The underwater robot passes through the gate without touching it. ", ""], ["19", "A3: Underwater", "", "The underwater robot passes through the gate within the first 30 minutes from the start of the run. ", ""], ["20", "A3: Underwater", "", "The underwater robot detects the five plume buoys in real time. Images are needed. ", ""], ["21", "A3: Underwater", "", "The underwater robot recognises the number on the five plume buoys. ", ""], ["22", "A3: Underwater", "", "The underwater robot produces a geometric map of the plume (Area: B1+B2). Father area from\nthe piping assembly", ""], ["23", "A3: Underwater", "", "The underwater robot produces a geometric map of the plume (Area: B3+B4+B5). Closer area to\nthe pipping assembly", ""], ["24", "A3: Underwater", "", "The underwater robot inspects the 4 pipes underwater. ", ""], ["25", "A3: Underwater", "", "The underwater robot detects the leak marker on the pipe in real time. ", ""], ["26", "A3: Underwater", "", "The underwater robot reports which is the number of the leaking pipe by its geometric position. ", ""], ["27", "A3: Underwater", "", "The underwater robot recognises and provides images of the black number stamped on the leaking\npipe", ""], ["28", "A3: Underwater", "", "Following the leaking pipe up to the assembly structure, the underwater robot provides an image\nmosaic of the first half of the leaking pipe. ", ""], ["29", "A3: Underwater", "", "Following the leaking pipe up to the assembly structure, the underwater robot provides an image\nmosaic of the second half of the leaking pipe. ", ""], ["30", "A3: Underwater", "", "The underwater robot provides a 3D reconstruction of the manipulation console where the correct\nunderwater valve is. ", ""], ["31", "A3: Underwater", "", "The underwater robot closes the correct valve with a rotation of the first 45 degrees. The process\nmust be recorded by the on board camera of the robot. ", ""], ["32", "A3: Underwater", "", "The underwater robot closes the correct valve with a rotation of the last 45 degrees (the process\nmust be recorded by the on board camera of the robot).", ""], ["33", "A4: Cooperation", "", "The underwater robot communicates through a surface robot or directly to the ground robot the\nfound leaking pipe.", ""], ["34", "A4: Cooperation", "", "The ground robot receives and decodes the message with the correct leaking pipe sent by directly\nby the underwater or through the surface robot. ", ""], ["35", "A4: Cooperation", "", "The ground robot communicates the correct land leaking pipe to the underwater robot (directly or\nthrough the surface robot). ", ""], ["36", "A4: Cooperation", "", "The underwater robot receives and decodes the message with the correct land leaking pipe sent by\nthe ground robot or the surface robot", ""], ["37", "A4: Cooperation", "", "The ground robot and the underwater robot close the correct valves in a synchronised process.", ""]]  # TBM 4
      (unwired) T4 [{"String"="Underwater 1 Plume (made of 5 orange buoys)", "Value"=0}, {"String"="Underwater 1 Pipe leak", "Value"=1}, {"String"="Underwater Debris (4 objects)", "Value"=2}, {"String"="Underwater 1 gate (made of 2 orange buoys)", "Value"=3}, {"String"="outdoors first Pipe damages on land", "Value"=4}, {"String"="outdoors second Pipe damages on land", "Value"=5}, {"String"="outdoors third Pipe damages on land", "Value"=6}, {"String"="outdoors 1 Pipe leak on land", "Value"=7}, {"String"="general first  Missing Workers", "Value"=8}, {"String"="general second  Missing Workers", "Value"=9}]  # opi TBM3
      (unwired) T4 [{"String"="Outdoor - first blocked entrances", "Value"=1}, {"String"="Outdoor - second blocked entrances", "Value"=2}, {"String"="Outdoor - 1 unblocked entrance", "Value"=3}, {"String"="Outdoor - first damage on the wall", "Value"=4}, {"String"="Outdoor - second damage on the wall", "Value"=5}, {"String"="Outdoor - third damage on the wall", "Value"=6}, {"String"="indoor - 1 machine room entrance", "Value"=7}, {"String"="Indoor - first damage on the wall", "Value"=8}, {"String"="Indoor - second damage on the wall", "Value"=9}, {"String"="general - first missing workes", "Value"=10}, {"String"="general - second missing workers", "Value"=0}]  # opi TBM2
      (unwired) T4 [{"String"="Underwater - 1 plume (made of 5 orange buoys)", "Value"=1}, {"String"="Underwater - 1 pipe leaks", "Value"=2}, {"String"="Underwater - debris (4 objects)", "Value"=3}, {"String"="Underwater - 1 gate (made of 2 orange buoys)", "Value"=4}, {"String"="Outdoor - 1 Pipe leak on land", "Value"=5}, {"String"="Outdoor - first damages on the building wall", "Value"=6}, {"String"="Outdor - second damages on the building wall", "Value"=7}, {"String"="Outdoor - third damages on the building wall", "Value"=8}, {"String"="Indoor - 1 machine room entrance", "Value"=9}, {"String"="Indoor - 1 correct valve (of four valves)", "Value"=10}]  # opi TBM4
    }
    frame Enabled {
    }
  }
  n2 = Build Array (concatenate)("0", string[] ["out of list"] ("array"), "", w10, w10) -> (w14:string[])
  n3 = Build Array (concatenate)(w14, w3) -> (w4:string[][])
  n4 = control-ref of="Subtask"() -> (w23:refnum<vi>)
  n5 = control-ref of="Number registered subtask"() -> (w17:refnum<vi>)
  n6 = call "Aktualizacja listy z punktami do usunięcia -dane z dwoch kolumn.vi"("1 kolumna"=FALSE ("Kolmuny 1/2"), "text add 2"=3 ("index column name add"), "text add 1"=0, "Lista współrzędnych"=w4, "Lista z punktami do usunięcia"=w23) -> ()  [unwired: 7 in]
  n7 = call "confirm button.vi"() -> ()  [unwired: 5 in, 1 out]
  n8 = Obtain Notifier(name (unnamed)="Leaking pipe status", notification data type=T1 {"op"="publish", "topic"="common", "msg"={"sender_name"="", "receiver_name"="", "latitude"=0.0, "longitude"=0.0, "valve_number"=0, "status"=""}} ("Messages read 2")) -> (notifier out=w2:refnum<notifier>, error out=w1:errorcluster)  [unwired: 2 in, 1 out]
  n9 = call "Aktualizacja listy z punktami do usunięcia -dane z dwoch kolumn.vi"("Lista współrzędnych"=string[][] [] ("Subtask registered event"), "Lista z punktami do usunięcia"=w17) -> ()  [unwired: 10 in]
  n10 = while {
    shift-right: [w42] -> _
    shift-left: w4 -> [w27]
    shift-right: [w38] -> _
    shift-left: string[][] [] ("Subtask registered event") -> [w39]
    shift-right: [w34] -> _
    shift-left: string[][] [] ("Subtask registered event") -> [w35]
    tunnel: w2 -> [w33]
    tunnel: w1 -> [w32]
    tunnel: [w31] -> w8
    tunnel: [w30] -> w7
    shift-right: [w24] -> _
    shift-left: string[][] [["Underwater - 1 plume (made of 5 orange buoys)"], ["Underwater - 1 pipe leaks"], ["Underwater - debris (4 objects)"], ["Underwater - 1 gate (made of 2 orange buoys)"], ["Outdoor - 1 Pipe leak on land"], ["Outdoor - first damages on the building wall"], ["Outdor - second damages on the building wall"], ["Outdoor - third damages on the building wall"], ["Indoor - 1 machine room entrance"], ["Indoor - 1 correct valve (of four valves)"]] ("Subtask registered event 2") -> [w25]
    stop <- w37 stop-if-true
    # "Logowanie zdarzeń"
    n11 = event shown="[0] Timeout" {
      selector: _ -> [_ _ _ _ _ _ _ _ _ _]
      dyn-events: _ -> [_ _ _ _ _ _ _ _ _ _]
      timeout: 1000 -> [_ _ _ _ _ _ _ _ _ _]
      tunnel: w27 -> [w69 w96 w121 w141 w161 w185 w211 w236 w273 w322]
      tunnel: [w69 w94 w123 w141 w157 w184 w210 w236 w273 w322] -> w42
      tunnel: "Subtask" -> [_ w95 w122 _ w162 w189 w216 _ _ _]
      tunnel: [w66 w85 w114 w137 w152 w179 w207 w237 w272 w323] -> w38
      tunnel: w39 -> [w66 w88 w108 w138 w155 w182 w208 w237 w272 w323]
      tunnel: [_ _ _ _ _ _ _ _ _ "stop"] -> w37
      tunnel: "Mode" -> [_ w93 w120 _ w163 w190 w215 _ _ _]
      tunnel: w35 -> [w52 w92 w119 w144 w160 w188 w214 w235 w277 w326]
      tunnel: [w43 w92 w119 w144 w160 w188 w214 w234 w277 w326] -> w34
      tunnel: w33 -> [w73 w91 w118 w143 w159 w187 w213 w233 w276 w325]
      tunnel: w32 -> [w72 w90 w117 w142 w158 w186 w212 w232 w275 w324]
      tunnel: [w73 w91 w118 w143 w159 w187 w213 w231 w276 w325] -> w31
      tunnel: [w72 w90 w117 w142 w158 w186 w212 w230 w275 w324] -> w30
      tunnel: "List of robots" -> [_ w89 w109 _ w156 w183 w209 _ w274 _]
      tunnel: "Additional status" -> [_ w84 w113 _ w151 w177 w204 _ _ _]
      tunnel: w25 -> [w61 w83 w111 w136 w150 w175 w203 w229 w271 w321]
      tunnel: [w61 w83 w111 w136 w150 w175 w203 w229 w270 w321] -> w24
      event Timeout {
        n12 = event-data() -> ()  [unwired: 1 in, 1 out]
        n13 = global read "common msg from UAV-1.vi" "read messages from UAV-1"() -> (w51:T1)
        n14 = for {
          shift-right: [w80] -> w70
          shift-left: string[][] [] ("Subtask to do") -> [w81]
          tunnel: w69 -> [w75] mode=indexing
          n15 = Index Array(array=w75, index=2) -> (element=w74:string)
          n16 = Build Array (concatenate)(w81, w75) -> (w79:string[][])
          n17 = Equal?(x="Done", y=w74) -> (x = y?=w77:bool)
          n18 = Select(t=w81, s=w77, f=w79) -> (s? t:f=w80:string[][])
        }
        "Subtask to do" <- w70
        n19 = call "update status.vi"("read messages from AUV sparus in"=w51, "Subtask registered event in"=w52) -> ("zmiana statusu  nadawanaego do robota lub komunikatu do robota"=w49:bool, "read messages from AUV sparus out"=→"read messages from UAV-1":T1, "Subtask registered event out"=w48:T2[][])  [unwired: 6 in]
        n20 = global read "common msg.vi" "read messages common"() -> (w53:T1)
        n21 = Build Array (concatenate)(w52, w48) -> (w60:T2[][])
        n22 = Array Size(array=w66) -> (size(s)=w65:i32[])
        n23 = Select(t=w60, s=w49, f=w52) -> (s? t:f=w59:T2[][])
        n24 = call "update status.vi"("read messages from AUV sparus in"=w53, "Subtask registered event in"=w59) -> ("zmiana statusu  nadawanaego do robota lub komunikatu do robota"=w58:bool, "read messages from AUV sparus out"=→"read messages from AUV sparus":T1, "Subtask registered event out"=w43:T2[][])  [unwired: 6 in]
        n25 = Index Array(array=w65, index=0) -> (element=w64:i32)
        n26 = Or(x=w58, y=w49) -> (x .or. y?=w56:bool)
        n27 = Array Subset(array=w66, length (row)=w64, index (col)=1 ("index 2"), length (col)=7 ("length 2")) -> (w62:T5[][])  [unwired: 1 in]
        n28 = call "Elapsed Time"("Reset"=w56) -> ("Time has Elapsed"=w57:bool)  [unwired: 11 in, 7 out]
        n29 = call "Zapis tabeli do pliku.vi"("2d array in"=w62) -> ("for 2d array out"=w46:string)  [unwired: 7 in, 1 out]
        n30 = Not(x=w57) -> (.not. x?=→"nowa wiadomość":bool)
        n31 = call "Zapis tabeli do pliku.vi"("2d array in"=w43) -> ("for 2d array out"=w44:string)  [unwired: 7 in, 1 out]
        n32 = Write to Text File(file (use dialog)="Subtask registered eveny", text=w46) -> ()  [unwired: 2 in, 3 out]
        n33 = Write to Text File(file (use dialog)="Status sent between robots", text=w44) -> ()  [unwired: 2 in, 3 out]
      }
      event "Setup": Value Change {
        n34 = event-data() -> ()  [unwired: 1 in, 1 out]
        n35 = call "confirm button.vi"() -> ("T button?"=w82:bool)  [unwired: 5 in]
        n36 = case shown="True" w82 {
          tunnel: w96 -> [w97 w107]
          tunnel: w95 -> [_ w106]
          tunnel: [w97 w105] -> w94
          tunnel: w93 -> [_ w104]
          tunnel: w89 -> [_ w103]
          tunnel: w88 -> [w98 w102]
          tunnel: [w98 w101] -> w85
          tunnel: w84 -> [_ w100]
          frame False {
          }
          frame True {
            n37 = call "add event.vi"("Mode"=w104, "TBM 5"=w107, "Subtask"=w106, "Combo Box"=T5 "Setup", "Additional info"=w100, "List of robots"=w103, "Subtask registered event in"=w102) -> ("Subtask registered event out"=w101:T5[][], "TBM 4"=w105:string[][])  [unwired: 11 in]
          }
        }
        n38 = control-ref of="Number registered subtask"() -> (w87:refnum<vi>)
        n39 = call "Aktualizacja listy z punktami do usunięcia -dane z dwoch kolumn.vi"("text add 1"=0, "Lista współrzędnych"=w85, "Lista z punktami do usunięcia"=w87) -> ()  [unwired: 9 in]
      }
      event "Ready": Value Change {
        n40 = event-data() -> ()  [unwired: 1 in, 1 out]
        n41 = call "confirm button.vi"() -> ("T button?"=w110:bool)  [unwired: 5 in]
        n42 = case shown="False" w110 {
          tunnel: [w125 w134] -> w123
          tunnel: w122 -> [_ w133]
          tunnel: w121 -> [w125 w132]
          tunnel: w120 -> [_ w131]
          tunnel: [w124 w130] -> w114
          tunnel: w113 -> [_ w129]
          tunnel: T5 "Ready" ("Combo Box") -> [_ w128]
          tunnel: w109 -> [_ w127]
          tunnel: w108 -> [w124 w126]
          frame False {
          }
          frame True {
            n43 = call "add event.vi"("Mode"=w131, "TBM 5"=w132, "Subtask"=w133, "Combo Box"=w128, "Additional info"=w129, "List of robots"=w127, "Subtask registered event in"=w126) -> ("Subtask registered event out"=w130:T5[][], "TBM 4"=w134:string[][])  [unwired: 11 in]
          }
        }
        n44 = control-ref of="Number registered subtask"() -> (w116:refnum<vi>)
        n45 = call "Aktualizacja listy z punktami do usunięcia -dane z dwoch kolumn.vi"("text add 1"=0, "Lista współrzędnych"=w114, "Lista z punktami do usunięcia"=w116) -> ()  [unwired: 9 in]
      }
      event "Delete": Value Change {
        n46 = event-data() -> ()  [unwired: 1 in, 1 out]
        n47 = call "confirm button.vi"() -> ("T button?"=w135:bool)  [unwired: 5 in]
        n48 = case shown="True" w135 {
          tunnel: w138 -> [w145 w147]
          tunnel: [w145 w146] -> w137
          frame False {
          }
          frame True {
            n49 = control-ref of="Number registered subtask"() -> (w148:refnum<vi>)
            n50 = call "Usuwanie punktu z listy współrzędnych.vi"("Lista współrzędnych"=w147, "Lista z punktami do usunięcia"=w148) -> ("Lista współrzędnych 2"=w146:string[][])  [unwired: 9 in]
          }
        }
        n51 = control-ref of="Number registered subtask"() -> (w140:refnum<vi>)
        n52 = call "Aktualizacja listy z punktami do usunięcia -dane z dwoch kolumn.vi"("text add 1"=0, "Lista współrzędnych"=w137, "Lista z punktami do usunięcia"=w140) -> ()  [unwired: 9 in]
      }
      event "Start": Value Change {
        n53 = event-data() -> ()  [unwired: 1 in, 1 out]
        n54 = call "confirm button.vi"() -> ("T button?"=w149:bool)  [unwired: 5 in]
        n55 = case shown="True" w149 {
          tunnel: w163 -> [_ w174]
          tunnel: w162 -> [_ w173]
          tunnel: w161 -> [w164 w172]
          tunnel: [w164 w171] -> w157
          tunnel: w156 -> [_ w170]
          tunnel: w155 -> [w165 w169]
          tunnel: [w165 w168] -> w152
          tunnel: w151 -> [_ w166]
          frame False {
          }
          frame True {
            n56 = call "add event.vi"("Mode"=w174, "TBM 5"=w172, "Subtask"=w173, "Combo Box"=T5 "Start", "Additional info"=w166, "List of robots"=w170, "Subtask registered event in"=w169) -> ("Subtask registered event out"=w168:T5[][], "TBM 4"=w171:string[][])  [unwired: 11 in]
          }
        }
        n57 = control-ref of="Number registered subtask"() -> (w154:refnum<vi>)
        n58 = call "Aktualizacja listy z punktami do usunięcia -dane z dwoch kolumn.vi"("text add 1"=0, "Lista współrzędnych"=w152, "Lista z punktami do usunięcia"=w154) -> ()  [unwired: 9 in]
      }
      event "Cancel": Value Change {
        n59 = event-data() -> ()  [unwired: 1 in, 1 out]
        n60 = call "confirm button.vi"() -> ("T button?"=w176:bool)  [unwired: 5 in]
        n61 = case shown="True" w176 {
          tunnel: w190 -> [_ w201]
          tunnel: w189 -> [_ w200]
          tunnel: w185 -> [w191 w199]
          tunnel: [w191 w198] -> w184
          tunnel: w183 -> [_ w197]
          tunnel: w182 -> [w192 w196]
          tunnel: [w192 w195] -> w179
          tunnel: T5 "Cancel" ("Combo Box") -> [_ w194]
          tunnel: w177 -> [_ w193]
          frame False {
          }
          frame True {
            n62 = call "add event.vi"("Mode"=w201, "TBM 5"=w199, "Subtask"=w200, "Combo Box"=w194, "Additional info"=w193, "List of robots"=w197, "Subtask registered event in"=w196) -> ("Subtask registered event out"=w195:T5[][], "TBM 4"=w198:string[][])  [unwired: 11 in]
          }
        }
        n63 = control-ref of="Number registered subtask"() -> (w181:refnum<vi>)
        n64 = call "Aktualizacja listy z punktami do usunięcia -dane z dwoch kolumn.vi"("text add 1"=0, "Lista współrzędnych"=w179, "Lista z punktami do usunięcia"=w181) -> ()  [unwired: 9 in]
      }
      event "Done": Value Change {
        n65 = event-data() -> ()  [unwired: 1 in, 1 out]
        n66 = call "confirm button.vi"() -> ("T button?"=w202:bool)  [unwired: 5 in]
        n67 = case shown="True" w202 {
          tunnel: w216 -> [_ w227]
          tunnel: w215 -> [_ w226]
          tunnel: w211 -> [w217 w225]
          tunnel: [w217 w219] -> w210
          tunnel: w209 -> [_ w224]
          tunnel: w208 -> [w218 w223]
          tunnel: [w218 w222] -> w207
          tunnel: w204 -> [_ w221]
          frame False {
          }
          frame True {
            n68 = call "add event.vi"("Mode"=w226, "TBM 5"=w225, "Subtask"=w227, "Combo Box"=T5 "Done", "Additional info"=w221, "List of robots"=w224, "Subtask registered event in"=w223) -> ("Subtask registered event out"=w222:T5[][], "TBM 4"=w219:string[][])  [unwired: 11 in]
          }
        }
        n69 = control-ref of="Number registered subtask"() -> (w206:refnum<vi>)
        n70 = call "Aktualizacja listy z punktami do usunięcia -dane z dwoch kolumn.vi"("text add 1"=0, "Lista współrzędnych"=w207, "Lista z punktami do usunięcia"=w206) -> ()  [unwired: 9 in]
      }
      event "Add leaking pipe": Value Change {
        n71 = event-data() -> ()  [unwired: 1 in, 1 out]
        n72 = call "confirm button.vi"() -> ("T button?"=w228:bool)  [unwired: 5 in]
        n73 = case shown="True" w228 {
          tunnel: w235 -> [w240 w262]
          tunnel: [w240 w261] -> w234
          tunnel: w233 -> [w239 w253]
          tunnel: w232 -> [w238 w251]
          tunnel: [w239 w254] -> w231
          tunnel: [w238 w255] -> w230
          frame False {
          }
          frame True {
            n74 = call "UTC KML time.vi"() -> ("String"=w256:string)  [unwired: 19 in]
            n75 = case shown="\"UGV2-Quadron\", Default" "sender robot" {
              tunnel: [w264 w266] -> w242
              tunnel: [w263 w265] -> w241
              frame "UGV2-Quadron", Default {
                n76 = global read "longitude Quadron.vi" "Longitude Quadron"() -> (w263:dbl)
                n77 = global read "latitude Quadron.vi" "latitude Quadron"() -> (w264:dbl)
              }
              frame "UGV1-Raptor" {
                n78 = global read "latitude.vi" "latitude"() -> (w266:dbl)
                n79 = global read "longitude.vi" "Longitude"() -> (w265:dbl)
              }
            }
            n80 = Number To Fractional String(number=w242) -> (F-format string=w259:string)  [unwired: 3 in]
            n81 = Number To Fractional String(number=w241) -> (F-format string=w258:string)  [unwired: 3 in]
            n82 = Number To Decimal String(number="Pipe") -> (decimal integer string=w257:string)  [unwired: 1 in]
            n83 = Build Array("sender robot", "receiver robot", w259, w258, w257, "Status", w256) -> (w260:T2[])
            n84 = Select(t="String", s="Mode 3", f="Status") -> (s? t:f=w244:T2)
            n85 = Bundle By Name(cluster=T1 {"op"="publish", "topic"="common", "msg"={"sender_name"="", "receiver_name"="", "latitude"=0.0, "longitude"=0.0, "valve_number"=0, "status"=""}} ("Messages read"), "msg.sender_name"="sender robot", "msg.receiver_name"="receiver robot", "msg.latitude"=w242, "msg.longitude"=w241, "msg.valve_number"="Pipe", "msg.status"=w244) -> (w252:T1)
            n86 = Build Array (concatenate)(w262, w260) -> (w261:T2[][])
            n87 = Send Notification(notification=w252, notifier=w253, error in (no error)=w251) -> (notifier out=w254:refnum<notifier>, error out=w255:errorcluster)
          }
        }
      }
      event "found": Value Change {
        n88 = event-data() -> ()  [unwired: 1 in, 1 out]
        n89 = call "confirm button.vi"() -> ("T button?"=w267:bool)  [unwired: 5 in]
        n90 = control-ref of="OPI to find"() -> ()  [unwired: 1 out]
        n91 = case shown="True" w267 {
          tunnel: w274 -> [_ w300]
          tunnel: w271 -> [w278 w296]
          tunnel: [w278 w298] -> w270
          tunnel: "Mode 2" -> [_ w290]
          tunnel: "Additional found item" -> [_ w292]
          frame False {
          }
          frame True {
            n92 = case shown="\"UAV-2\"" w300 {
              tunnel: [_ w312 w313 w316 w318 w320] -> w302
              tunnel: [_ w311 w314 w315 w317 w319] -> w303
              frame "False", Default {
              }
              frame "UGV1-Raptor" {
                n93 = global read "longitude.vi" "Longitude"() -> (w312:dbl)
                n94 = global read "latitude.vi" "latitude"() -> (w311:dbl)
              }
              frame "AUV-Sparus" {
                n95 = global read "Longitude Sparus.vi" "Longitude Sparus"() -> (w314:dbl)
                n96 = global read "Latitude Sparus.vi" "Latitude Sparus"() -> (w313:dbl)
              }
              frame "UGV2-Quadron" {
                n97 = global read "longitude Quadron.vi" "Longitude Quadron"() -> (w315:dbl)
                n98 = global read "latitude Quadron.vi" "latitude Quadron"() -> (w316:dbl)
              }
              frame "UAV-1" {
                n99 = global read "Longitude dron 1.vi" "Longitude dron 1"() -> (w317:dbl)
                n100 = global read "Latitude dron 1.vi" "Latitude dron 1"() -> (w318:dbl)
              }
              frame "UAV-2" {
                n101 = global read "Longitude dron 2.vi" "Longitude dron 2"() -> (w319:dbl)
                n102 = global read "Latitude dron 2.vi" "Latitude dron 2"() -> (w320:dbl)
              }
            }
            n103 = call "UTC KML time.vi"() -> ("String"=w305:string)  [unwired: 19 in]
            n104 = control-ref of="OPI to find"() -> (w299:refnum<vi>)
            n105 = case shown="True" w290 {
              tunnel: w299 -> [w309 _]
              tunnel: [w308 w310] -> w298
              tunnel: w296 -> [w306 w310]
              frame False {
                n106 = call "Usuwanie punktu z listy współrzędnych.vi"("Aktywacja potwierdzenia"=FALSE, "Lista współrzędnych"=w306, "Lista z punktami do usunięcia"=w309) -> ("Lista współrzędnych 2"=w308:string[][])  [unwired: 8 in]
                n107 = call "Aktualizacja listy z punktami do usunięcia -dane z dwoch kolumn.vi"("Lista współrzędnych"=w308, "Lista z punktami do usunięcia"=w309) -> ()  [unwired: 10 in]
              }
              frame True {
              }
            }
            n108 = Number To Fractional String(number=w302) -> (F-format string=w301:string)  [unwired: 3 in]
            n109 = Number To Fractional String(number=w303) -> (F-format string=w297:string)  [unwired: 3 in]
            n110 = Decrement(x="OPI to find") -> (x-1=w294:u16)
            n111 = Index Array(array=w296, index (row)=w294, index (col)=0 ("disabled index (col)")) -> (element=w291:string)
            n112 = Select(t=w292, s=w290, f=w291) -> (s? t:f=w288:string)
            n113 = Concatenate Strings(w288, " " ("string"), "target ID") -> (w289:string)
            n114 = Build Array(w305, w289, w301, w297, "... .jpg", w300) -> (w282:T2[])
            n115 = Read from Text File(file (use dialog)="Object recognition") -> (text=w285:string)  [unwired: 3 in, 3 out]
            n116 = local write "Additional status"(w289) -> ()
            n117 = Concatenate Strings(w285, w282) -> (w284:string)
            n118 = Write to Text File(file (use dialog)="Object recognition", text=w284) -> ()  [unwired: 2 in, 3 out]
            n119 = feedback #1(T2[][] []) -> (w281:T2[][])
            n120 = Build Array (concatenate)(w281, w282) -> (w280:T2[][])
            "OPI found" <- w280
            n121 = feedback-in #1(w280) -> ()
          }
        }
      }
      event "stop": Value Change {
        n122 = event-data() -> ()  [unwired: 1 in, 1 out]
      }
    }
    "All Subtask Status" <- w42
    "Subtask registered event" <- w38
    "Status sent between robots and control station" <- w34
    n123 = Wait Until Next ms Multiple(millisecond multiple=u32 10) -> ()  [unwired: 1 out]
  }
  n124 = while {
    tunnel: w2 -> [w330]
    tunnel: w1 -> [w329]
    stop <- FALSE stop-if-true
    # "Wysyłanie do  ROS-a drone 1"
    n125 = Wait Until Next ms Multiple(millisecond multiple=u32 1000 ("milliseconds to wait")) -> ()  [unwired: 1 out]
    n126 = case shown="True" "ROSB WRITE 2" {
      tunnel: w330 -> [_ w334]
      tunnel: w329 -> [_ w333]
      frame False {
      }
      frame True {
        n127 = TCP Open Connection(address="rosbridge server IP 3", remote port or service name="rosbridge port 3") -> (connection ID=w338:refnum<k5>, error out=w337:errorcluster)  [unwired: 3 in]
        n128 = TCP Write(connection ID=w338, data in="GET / HTTP/1.1\nUpgrade: websocket\nConnection: Upgrade\nHost: 192.168.5.103:9090\nOrigin: http://192.168.5.101:9090\nSec-WebSocket-Key: pM4mFvl5nUXJXjxIa41LvQ==\nSec-WebSocket-Version: 13", error in (no error)=w337) -> (connection ID out=w336:refnum<k5>, error out=w335:errorcluster)  [unwired: 1 in, 1 out]
        n129 = call <vilib>:"Write.vi"("error in (no error)"=w335, "Data"="advertise msg 3", "WebSocket Connection in"=w336) -> ("error out"=w353:errorcluster, "WebSocket Connection out"=w354:refnum<k5>)  [unwired: 7 in]
        n130 = while {
          tunnel: [w364] -> w346
          tunnel: [w357] -> w345
          tunnel: w354 -> [w365]
          tunnel: w353 -> [w366]
          tunnel: w334 -> [w362]
          tunnel: w333 -> [w361]
          stop <- w355 stop-if-true
          n131 = Get Notifier Status(notifier=w362, error in (no error)=w361) -> (current notification=w359:T1)  [unwired: 4 out]
          "sent messages  2" <- w359
          n132 = Unbundle By Name(w359) -> ("op"=w358:string)
          n133 = Empty String/Path?(string/path=w358) -> (empty?=w360:bool)
          n134 = case shown="True" w360 {
            tunnel: w366 -> [w373 w374]
            tunnel: w365 -> [w372 w375]
            tunnel: [w371 w375] -> w364
            tunnel: [w368 w374] -> w357
            tunnel: w359 -> [w367 _]
            frame False {
              n135 = Flatten To JSON(anything=w367, error in (no error)=w373) -> (JSON string=w369:string, 11:w370:errorcluster)  [unwired: 1 in]
              "raw frame 5" <- w369
              n136 = call <vilib>:"Write.vi"("error in (no error)"=w370, "Data"=w369, "WebSocket Connection in"=w372) -> ("error out"=w368:errorcluster, "WebSocket Connection out"=w371:refnum<k5>)  [unwired: 7 in]
            }
            frame True {
            }
          }
          n137 = Wait (ms)(milliseconds to wait=u32 1000) -> ()  [unwired: 1 out]
          n138 = Or(x=w357, y="STOP ROS WRITE 2") -> (x .or. y?=w355:bool)
        }
        n139 = Search and Replace String(input string="advertise msg 3", search string="advertise", replace string="unadvertise" ("search string")) -> (result string=w341:string)  [unwired: 5 in, 3 out]
        n140 = call <vilib>:"Write.vi"("error in (no error)"=w345, "Data"=w341, "WebSocket Connection in"=w346) -> ("error out"=w347:errorcluster, "WebSocket Connection out"=w348:refnum<k5>)  [unwired: 7 in]
        n141 = call <vilib>:"Close.vi"("error in (no error)"=w347, "WebSocket Connection in"=w348) -> ("error out"=w351:errorcluster, "WebSocket Connection in"=w350:refnum<k5>)  [unwired: 8 in]
        n142 = TCP Close Connection(connection ID=w350, error in (no error)=w351) -> (error out=→"error out 5":errorcluster)  [unwired: 1 in, 1 out]
      }
    }
  }
  n143 = while {
    tunnel: w2 -> [w378]
    tunnel: w1 -> [w377]
    stop <- FALSE stop-if-true
    # "Wysyłanie do ROS-a Sparus"
    n144 = Wait Until Next ms Multiple(millisecond multiple=u32 1000 ("milliseconds to wait")) -> ()  [unwired: 1 out]
    n145 = case shown="True" "ROSB WRITE" {
      tunnel: w378 -> [_ w382]
      tunnel: w377 -> [_ w381]
      frame False {
      }
      frame True {
        n146 = TCP Open Connection(address="rosbridge server IP 2", remote port or service name="rosbridge port 2") -> (connection ID=w386:refnum<k5>, error out=w385:errorcluster)  [unwired: 3 in]
        n147 = TCP Write(connection ID=w386, data in="GET / HTTP/1.1\nUpgrade: websocket\nConnection: Upgrade\nHost: 192.168.5.103:9090\nOrigin: http://192.168.5.101:9090\nSec-WebSocket-Key: pM4mFvl5nUXJXjxIa41LvQ==\nSec-WebSocket-Version: 13", error in (no error)=w385) -> (connection ID out=w384:refnum<k5>, error out=w383:errorcluster)  [unwired: 1 in, 1 out]
        n148 = call <vilib>:"Write.vi"("error in (no error)"=w383, "Data"="advertise msg 2", "WebSocket Connection in"=w384) -> ("error out"=w401:errorcluster, "WebSocket Connection out"=w402:refnum<k5>)  [unwired: 7 in]
        n149 = while {
          tunnel: [w412] -> w394
          tunnel: [w405] -> w393
          tunnel: w402 -> [w413]
          tunnel: w401 -> [w414]
          tunnel: w382 -> [w410]
          tunnel: w381 -> [w409]
          stop <- w403 stop-if-true
          n150 = Get Notifier Status(notifier=w410, error in (no error)=w409) -> (current notification=w407:T1)  [unwired: 4 out]
          "sent messages" <- w407
          n151 = Unbundle By Name(w407) -> ("op"=w406:string)
          n152 = Empty String/Path?(string/path=w406) -> (empty?=w408:bool)
          n153 = Wait (ms)(milliseconds to wait=u32 1000) -> ()  [unwired: 1 out]
          n154 = case shown="False" w408 {
            tunnel: w414 -> [w421 w422]
            tunnel: w413 -> [w420 w423]
            tunnel: [w419 w423] -> w412
            tunnel: [w416 w422] -> w405
            tunnel: w407 -> [w415 _]
            frame False {
              n155 = Flatten To JSON(anything=w415, error in (no error)=w421) -> (JSON string=w417:string, 11:w418:errorcluster)  [unwired: 1 in]
              "raw frame 4" <- w417
              n156 = call <vilib>:"Write.vi"("error in (no error)"=w418, "Data"=w417, "WebSocket Connection in"=w420) -> ("error out"=w416:errorcluster, "WebSocket Connection out"=w419:refnum<k5>)  [unwired: 7 in]
            }
            frame True {
            }
          }
          n157 = Or(x=w405, y="STOP ROS WRITE") -> (x .or. y?=w403:bool)
        }
        n158 = Search and Replace String(input string="advertise msg 2", search string="advertise", replace string="unadvertise" ("search string")) -> (result string=w389:string)  [unwired: 5 in, 3 out]
        n159 = call <vilib>:"Write.vi"("error in (no error)"=w393, "Data"=w389, "WebSocket Connection in"=w394) -> ("error out"=w395:errorcluster, "WebSocket Connection out"=w396:refnum<k5>)  [unwired: 7 in]
        n160 = call <vilib>:"Close.vi"("error in (no error)"=w395, "WebSocket Connection in"=w396) -> ("error out"=w399:errorcluster, "WebSocket Connection in"=w398:refnum<k5>)  [unwired: 8 in]
        n161 = TCP Close Connection(connection ID=w398, error in (no error)=w399) -> (error out=→"error out 4":errorcluster)  [unwired: 1 in, 1 out]
      }
    }
  }
  n162 = Release Notifier(notifier=w8, error in (no error)=w7) -> (error out=w6:errorcluster)  [unwired: 1 in, 2 out]
  n163 = call <vilib>:"Simple Error Handler.vi"("error in (no error)"=w6) -> ()  [unwired: 4 in, 5 out]
